vi "Time_I-V_Spliter.vi"(0 "DataFile":string[][](array[string])=array63093x51[3217743 elements], 1 "Real Time scale":bool) -> (2 "Time":timestamp[](array[timestamp]), 3 "Current":T1, 4 "Voltage":T1)   [LabVIEW 2018]
uses:
  <vilib>/Analysis/Matrix/Datatypes/RealMatrix.ctl
  <vilib>/Analysis/Matrix/NI_Matrix.lvlib
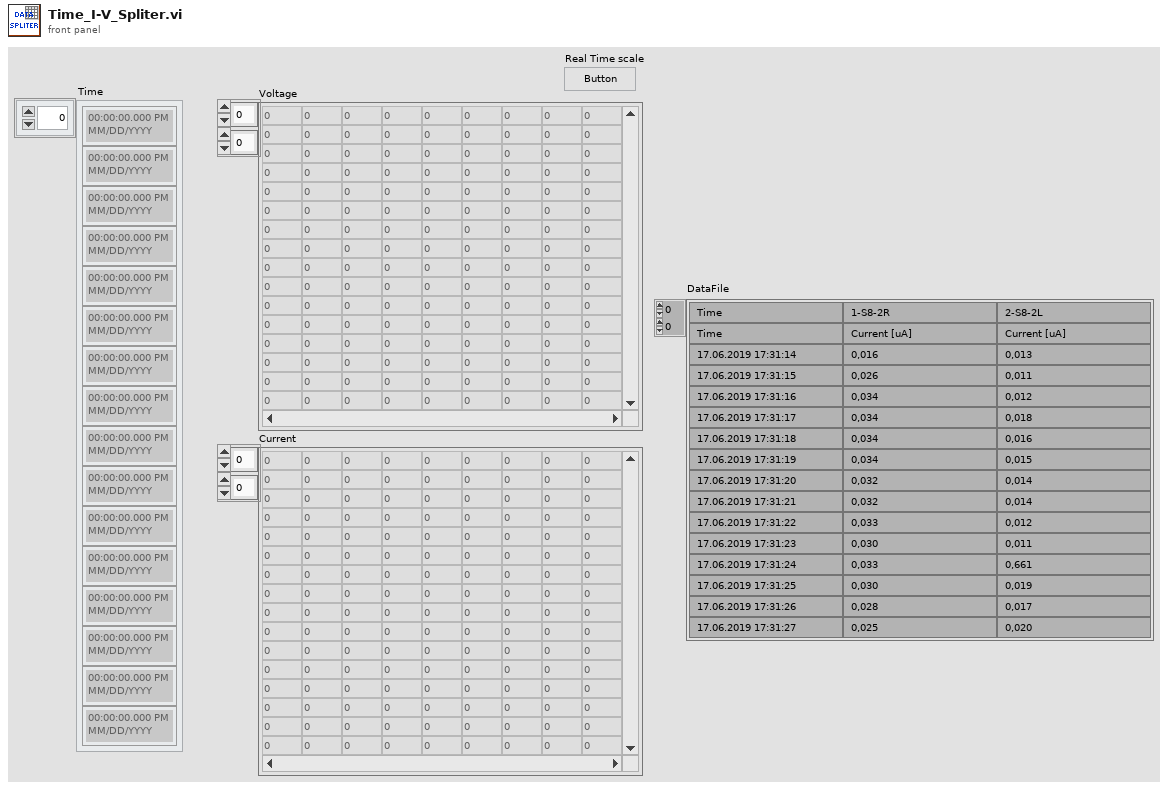
[diagram p1: front panel]
types:
  T1 = typedef "NI_Matrix.lvlib/RealMatrix.ctl" = dbl[][]
  T2 = typedef "LVDateTimeRec.ctl" = cluster{"fractional second":dbl, "second":i32, "minute":i32, "hour":i32, "day of month":i32, "month":i32, "year":i32, "day of week":i32, "day of year":i32, "DST":i32}
  T3 = cluster{dbl, i32, i32, i32, "day of month":i32, "month":i32, "year":i32, "day of week":i32, "day of year":i32, "DST":i32}
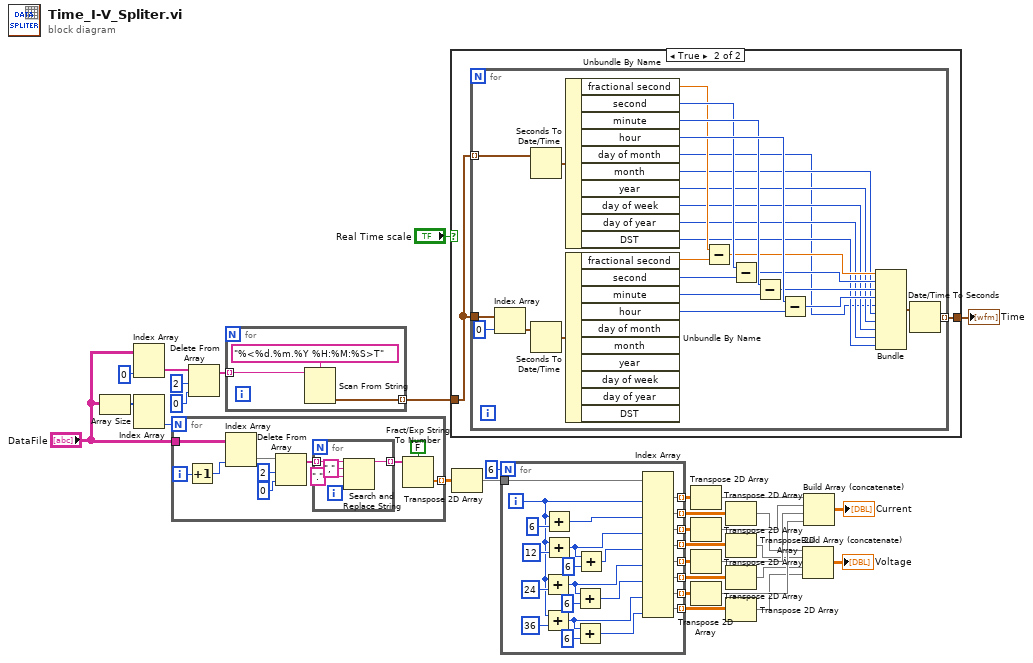
[diagram p0: block diagram]
diagram:
  n1 = Array Size(array="DataFile") -> (size(s)=w28:i32[])
  n2 = Index Array(array="DataFile", index (col)=0 ("disabled index (col)")) -> (element=w29:string[])  [unwired: 1 in]
  n3 = Index Array(array=w28) -> (element #2=w1:i32)  [unwired: 2 in, 1 out]
  n4 = for {
    N: w1 -> [_]
    tunnel: "DataFile" -> [w39]
    tunnel: [w38] -> w27 mode=indexing
    i -> [w35]
    n5 = Increment(x=w35) -> (x+1=w34:i32)
    n6 = Index Array(array=w39, index (col)=w34) -> (element=w42:string[])  [unwired: 1 in]
    n7 = Delete From Array(array=w42, length=2, index=0) -> (array with subset deleted=w37:string[])  [unwired: 1 out]
    n8 = for {
      tunnel: w37 -> [w44] mode=indexing
      tunnel: [w43] -> w36 mode=indexing
      n9 = Search and Replace String(input string=w44, search string=",", replace string="." ("replace string (\"\")")) -> (result string=w43:string)  [unwired: 5 in, 3 out]
    }
    n10 = Fract/Exp String To Number(use system decimal point (T)=FALSE, string=w36) -> (number=w38:dbl[])  [unwired: 2 in, 1 out]
  }
  n11 = Delete From Array(array=w29, length=2, index=0) -> (array with subset deleted=w5:string[])  [unwired: 1 out]
  n12 = for {
    tunnel: w5 -> [w48] mode=indexing
    tunnel: [w47] -> w4 mode=indexing
    n13 = Scan From String(format string="%<%d.%m.%Y %H:%M:%S>T", input string=w48) -> (output 1=w47:timestamp)  [unwired: 3 in, 3 out]
  }
  n14 = case shown="True" "Real Time scale" {
    tunnel: w4 -> [w50 w52]
    tunnel: [w50 w51] -> w3
    frame False {
    }
    frame True {
      n15 = for {
        tunnel: w52 -> [w65] mode=indexing
        tunnel: [w64] -> w51 mode=indexing
        tunnel: w52 -> [w62]
        n16 = Index Array(array=w62, index=0) -> (element=w63:timestamp)
        n17 = Seconds To Date/Time(time stamp (now)=w65) -> (date time rec=w75:T2)  [unwired: 1 in]
        n18 = Seconds To Date/Time(time stamp (now)=w63) -> (date time rec=w66:T2)  [unwired: 1 in]
        n19 = Unbundle By Name(w75) -> ("fractional second"=w74:dbl, "second"=w76:i32, "minute"=w77:i32, "hour"=w78:i32, "day of month"=w53:i32, "month"=w59:i32, "year"=w58:i32, "day of week"=w56:i32, "day of year"=w55:i32, "DST"=w54:i32)
        n20 = Unbundle By Name(w66) -> ("fractional second"=w67:dbl, "second"=w68:i32, "minute"=w69:i32, "hour"=w70:i32)  [unwired: 6 out]
        n21 = Subtract(x=w74, y=w67) -> (x-y=w71:dbl)
        n22 = Subtract(x=w76, y=w68) -> (x-y=w72:i32)
        n23 = Subtract(x=w77, y=w69) -> (x-y=w73:i32)
        n24 = Subtract(x=w78, y=w70) -> (x-y=w60:i32)
        n25 = Bundle(w71, w72, w73, w60, "day of month"=w53, "month"=w59, "year"=w58, "day of week"=w56, "day of year"=w55, "DST"=w54) -> (w57:T3)  [unwired: 1 in]
        n26 = Date/Time To Seconds(2:w57) -> (0:w64:timestamp)  [unwired: 1 in]
      }
    }
  }
  "Time" <- w3
  n27 = Transpose 2D Array(2D array=w27) -> (transposed array=w24:dbl[][])
  n28 = for {
    N: 6 -> [_]
    tunnel: w24 -> [w95]
    tunnel: [w86] -> w19 mode=indexing
    tunnel: [w85] -> w23 mode=indexing
    tunnel: [w84] -> w18 mode=indexing
    tunnel: [w83] -> w22 mode=indexing
    tunnel: [w82] -> w17 mode=indexing
    tunnel: [w81] -> w21 mode=indexing
    tunnel: [w80] -> w16 mode=indexing
    tunnel: [w79] -> w20 mode=indexing
    i -> [w94]
    n29 = Add(x=w94, y=24) -> (x+y=w90:i32)
    n30 = Add(x=w94, y=36) -> (x+y=w88:i32)
    n31 = Add(x=w94, y=6) -> (x+y=w93:i32)
    n32 = Add(x=w94, y=12) -> (x+y=w92:i32)
    n33 = Add(x=w90, y=6) -> (x+y=w89:i32)
    n34 = Add(x=w88, y=6) -> (x+y=w87:i32)
    n35 = Add(x=w92, y=6) -> (x+y=w91:i32)
    n36 = Index Array(array=w95, index (col) #1=w94, index (col) #2=w93, index (col) #3=w92, index (col) #4=w91, index (col) #5=w90, index (col) #6=w89, index (col) #7=w88, index (col) #8=w87) -> (element #1=w86:dbl[], element #2=w85:dbl[], element #3=w84:dbl[], element #4=w83:dbl[], element #5=w82:dbl[], element #6=w81:dbl[], element #7=w80:dbl[], element #8=w79:dbl[])  [unwired: 8 in]
  }
  n37 = Transpose 2D Array(2D array=w19) -> (transposed array=w15:dbl[][])
  n38 = Transpose 2D Array(2D array=w18) -> (transposed array=w14:dbl[][])
  n39 = Transpose 2D Array(2D array=w17) -> (transposed array=w13:dbl[][])
  n40 = Transpose 2D Array(2D array=w16) -> (transposed array=w12:dbl[][])
  n41 = Transpose 2D Array(2D array=w23) -> (transposed array=w11:dbl[][])
  n42 = Transpose 2D Array(2D array=w22) -> (transposed array=w10:dbl[][])
  n43 = Transpose 2D Array(2D array=w21) -> (transposed array=w9:dbl[][])
  n44 = Transpose 2D Array(2D array=w20) -> (transposed array=w8:dbl[][])
  n45 = Build Array (concatenate)(w11, w10, w9, w8) -> (→"Voltage":T1)
  n46 = Build Array (concatenate)(w15, w14, w13, w12) -> (→"Current":T1)
